vi "Create.vi"(8 "error in (no error)":errorcluster, 11 "Image":T1) -> (0 "error out":errorcluster, 3 "Camera Data":refnum<data-value>)   [LabVIEW 2022 SP3, in "Camera Data.lvclass"]
uses:
  Camera Data.lvclass
  <vilib>/vision/Image Controls.llb/IMAQ Image.ctl
  Camera Data.lvclass/Camera Data.ctl
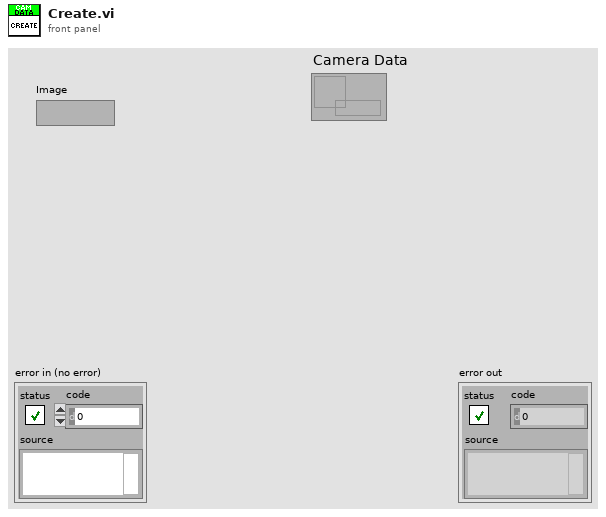
[diagram p1: front panel]
types:
  T1 = typedef "IMAQ Image.ctl" = refnum<image>
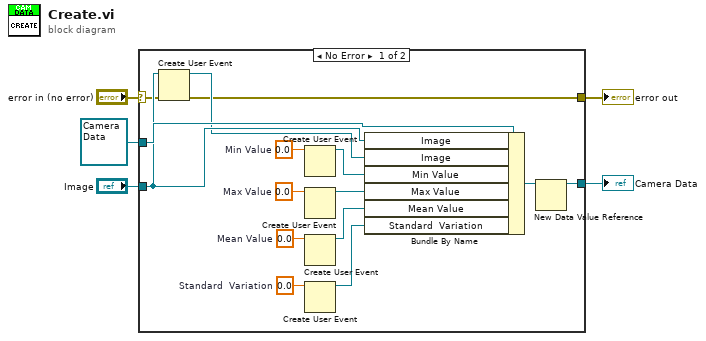
[diagram p0: block diagram]
diagram:
  n1 = case shown="No Error" "error in (no error)" {
    selector: "error in (no error)" -> [w17 w21]
    tunnel: [w16 w21] -> w4
    tunnel: refnum<class "Camera Data.lvclass"> refnum ("Camera Data in") -> [w20 _]
    tunnel: "Image" -> [w19 _]
    tunnel: [w14 _] -> w1
    frame No Error {
      w10 = sgl 0.0  # Standard  Variation
      w11 = sgl 0.0  # Mean Value
      w12 = 0.0  # Max Value
      w13 = 0.0  # Min Value
      n2 = Create User Event(user event datatype=w19, error in=w17) -> (user event=w18:refnum<user-event>, error out=w16:errorcluster)
      n3 = Create User Event(user event datatype=w13) -> (user event=w9:refnum<user-event>)  [unwired: 1 in, 1 out]
      n4 = Create User Event(user event datatype=w12) -> (user event=w8:refnum<user-event>)  [unwired: 1 in, 1 out]
      n5 = Create User Event(user event datatype=w11) -> (user event=w7:refnum<user-event>)  [unwired: 1 in, 1 out]
      n6 = Create User Event(user event datatype=w10) -> (user event=w6:refnum<user-event>)  [unwired: 1 in, 1 out]
      n7 = Bundle By Name(cluster=w20, "Image"=w19, "Image"=w18, "Min Value"=w9, "Max Value"=w8, "Mean Value"=w7, "Standard  Variation"=w6) -> (w15:refnum<class "Camera Data.lvclass">)
      n8 = New Data Value Reference(data value=w15) -> (data value reference=w14:refnum<data-value>)  [unwired: 1 in, 1 out]
    }
    frame Error {
    }
  }
  "error out" <- w4
  "Camera Data" <- w1
